vi "Sweep Control Inner Loop.vi"(8 "error in (no error)":errorcluster, 9 "inner loop index":i32, 10 "loop #":i32, 11 "SweepControl in":refnum<class "SMO.SweepControl.lvclass">) -> (0 "error out":errorcluster, 2 "Stop?":bool, 3 "SweepControl out":refnum<class "SMO.SweepControl.lvclass">)   [LabVIEW 2019, in "SMO.SweepControl.lvclass"]
uses:
  SMO.SweepControl.lvclass
  <userlib>/_OpenG.lib/array/array.llb/Empty 1D Array (Variant)__ogtk.vi
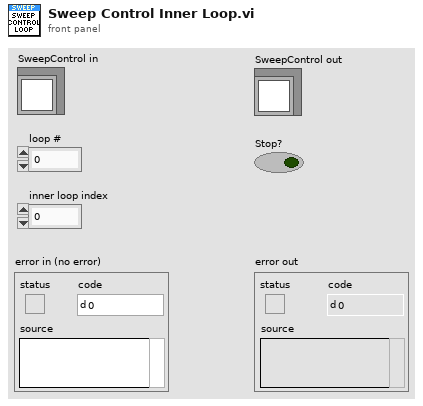
[diagram p1: front panel]
types:
  T1 = typedef "SMO.SweepControl.lvclass/ScanControl.ctl" = T2[]
  T2 = typedef "SMO.SweepControl.lvclass/Cluster - ScanControl.ctl" = cluster{"Priority":T3, "Scan name":T4}
  T3 = typedef "SMO.SweepControl.lvclass/Enum - Priority.ctl" = enum16{"Priority 0", "Priority 1", "Priority 2", "Priority 3", "Priority 4", "Priority 5"}
  T4 = typedef "SMO.SweepControl.lvclass/Enum - Action.ctl" = enum16{"OFF", "time", "Lockin Amplitude", "Lockin Frequency", "Lockin Bias", "Delay", "Strain", "DAQ Bias", "Magnet Field", "Temperature", "MW f1", "MW f2", "MW Amplitude1", "MW Amplitude2"}
  T5 = typedef "SMO.SweepControl.lvclass/PostAction.ctl" = T6[]
  T6 = typedef "SMO.SweepControl.lvclass/Enum - PostAction.ctl" = enum16{"Do Nothing", "Wait (time)", "Wait (Temperature)", "Wait (<T ; B sweep)", "Wait (Magnet)"}
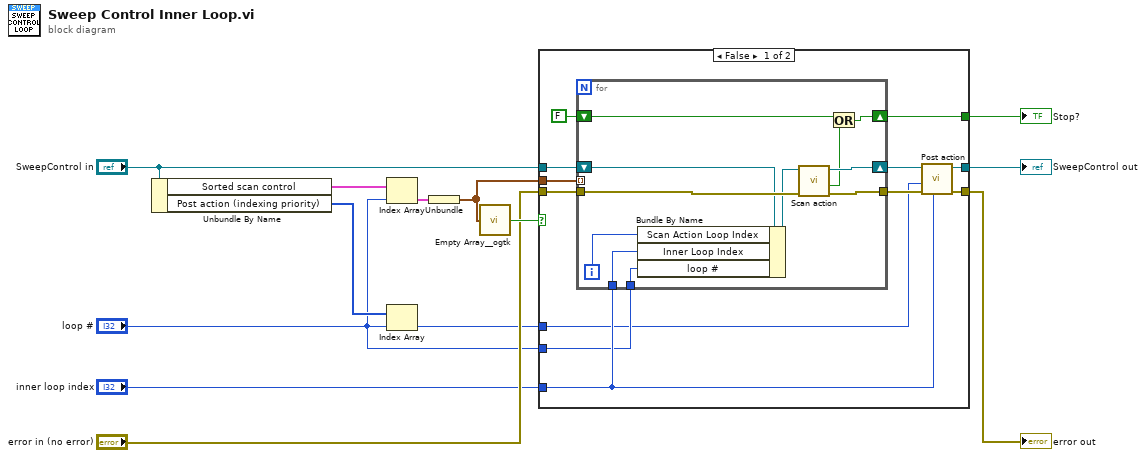
[diagram p0: block diagram]
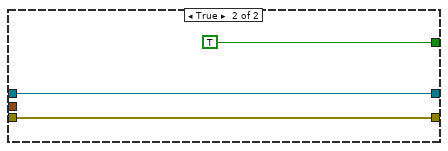
[diagram p2: hidden frame]
diagram:
  n1 = Unbundle By Name("SweepControl in") -> ("Sorted scan control"=w10:cluster{T1}[], "Post action (indexing priority)"=w9:T5)
  n2 = Index Array(array=w10, index="loop #") -> (element=w11:cluster{T1})
  n3 = Index Array(array=w9, index="loop #") -> (element=w5:T6)
  n4 = Unbundle(w11) -> (w4:T1)
  n5 = call-poly <userlib>:"Empty Array__ogtk.vi"("Array"=w4) -> ("Empty Array?"=w12:bool)  [unwired: 8 in]
  n6 = case shown="False" w12 {
    tunnel: [w24 TRUE ("Stop?")] -> w13
    tunnel: "loop #" -> [w18 _]
    tunnel: "error in (no error)" -> [w22 w38]
    tunnel: [w23 w38] -> w7
    tunnel: "inner loop index" -> [w20 _]
    tunnel: "SweepControl in" -> [w19 w37]
    tunnel: [w14 w37] -> w3
    tunnel: w5 -> [w17 _]
    tunnel: w4 -> [w16 _]
    frame False {
      n7 = for {
        shift-right: [w33] -> w24
        shift-left: FALSE -> [w36]
        tunnel: w22 -> [w35]
        tunnel: [w34] -> w21
        tunnel: w20 -> [w29]
        shift-right: [w32] -> w15
        shift-left: w19 -> [w27]
        tunnel: w18 -> [w28]
        tunnel: w16 -> [_] mode=indexing
        i -> [w30]
        n8 = Bundle By Name(cluster=w27, "Scan Action Loop Index"=w30, "Inner Loop Index"=w29, "loop #"=w28) -> (w26:refnum<class "SMO.SweepControl.lvclass">)
        n9 = call "Scan action.vi"("error in (no error)"=w35, "SweepControl in"=w26) -> ("error out"=w34:errorcluster, "Stop?"=w31:bool, "SweepControl out"=w32:refnum<class "SMO.SweepControl.lvclass">)  [unwired: 7 in]
        n10 = Or(x=w36, y=w31) -> (x .or. y?=w33:bool)
      }
      n11 = call "Post action.vi"("Index"=w20, "error in (no error)"=w21, "PostAction"=w17, "SweepControl"=w15) -> ("error out"=w23:errorcluster, "SweepControl"=w14:refnum<class "SMO.SweepControl.lvclass">)  [unwired: 6 in]
    }
    frame True {
    }
  }
  "SweepControl out" <- w3
  "Stop?" <- w13
  "error out" <- w7
